vi "ReadAcquisitionData.vi"(8 "error in (no error)":errorcluster, 9 "PicamAvailableData":T1, 11 "PicamHandle (camera)":u64) -> (0 "error out":errorcluster, 2 "DataAcquisitionBuffer out":T2, 3 "camera handle out":i64)   [LabVIEW 2019, in "PICam.lvlib"]
uses:
  PICam.lvlib
  types/utility/DataAcquisitionResult.ctl
  types/PicamRoi.ctl
  types/PicamAvailableData.ctl
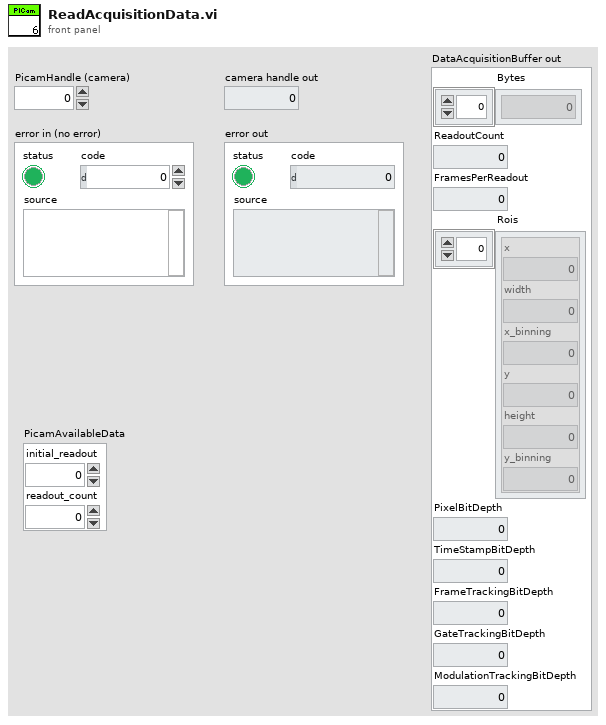
[diagram p1: front panel]
types:
  T1 = typedef "PicamAvailableData.ctl" = cluster{"initial_readout":u64, "readout_count":i64}
  T2 = typedef "DataAcquisitionResult.ctl" = cluster{"Bytes":u8[], "ReadoutCount":i64, "FramesPerReadout":i32, "Rois":T3[], "PixelBitDepth":i32, "TimeStampBitDepth":i32, "FrameTrackingBitDepth":i32, "GateTrackingBitDepth":i32, "ModulationTrackingBitDepth":i32}
  T3 = typedef "PicamRoi.ctl" = cluster{"x":i32, "width":i32, "x_binning":i32, "y":i32, "height":i32, "y_binning":i32}
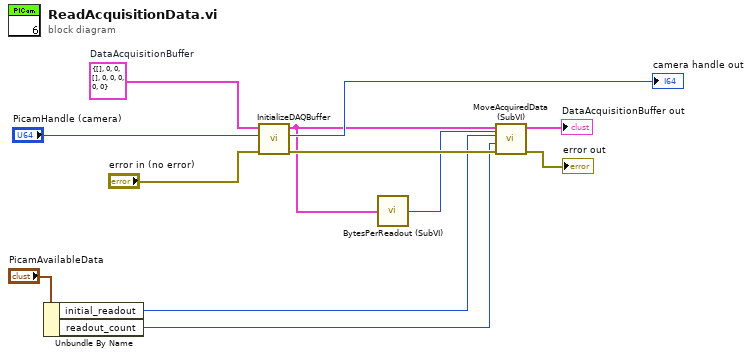
[diagram p0: block diagram]
diagram:
  w9 = T2 {"Bytes"=[], "ReadoutCount"=0, "FramesPerReadout"=0, "Rois"=[], "PixelBitDepth"=0, "TimeStampBitDepth"=0, "FrameTrackingBitDepth"=0, "GateTrackingBitDepth"=0, "ModulationTrackingBitDepth"=0}  # DataAcquisitionBuffer
  n1 = Unbundle By Name("PicamAvailableData") -> ("initial_readout"=w2:u64, "readout_count"=w1:i64)
  n2 = call "InitializeDAQBuffer.vi"("error in (no error)"="error in (no error)", "PicamHandle (camera)"="PicamHandle (camera)", "DataAcquisitionBuffer in"=w9) -> ("error out"=w10:errorcluster, "PicamHandle out"=→"camera handle out":u64, "DataAcquisitionBuffer out"=w7:T2)  [unwired: 6 in]
  n3 = call "BytesPerReadout (SubVI).vi"("DataAcquisitionBuffer in"=w7) -> ("Bytes/Readout >"=w5:i32)
  n4 = call "MoveAcquiredData (SubVI).vi"("Bytes/Readout >"=w5, "error in (no error)"=w10, "readout_count"=w1, "initial_readout*"=w2, "DataAcquisitionBuffer in"=w7) -> ("error out"=→"error out":errorcluster, "DataAcquisitionBuffer out"=→"DataAcquisitionBuffer out":T2)  [unwired: 5 in]
